vi "MMB.vi"() -> ()   [LabVIEW 2010]
doc: "INTRODUCTION:\nThis program will display a message on the moving message board display based on the user's input. It simulates a moving message board made up of an array of LED's or lights. The user can cause it to display a random pattern of Boolean LED's either turned off or on, a single Boolean LED point scrolling across the display from right to left, a scrolling column of Boolean LED's that can individually be turned on or off, or the message that is entered into the Message control. Any of these options can be repeated as many times as desired by toggling the \"Repeat\" Boolean Control. There is also a \"Milliseconds to Wait\" control, which adjusts the scrolling delay so that the scrolling looks smooth. Foreground and background colors can be changed via color box controls.\n\nDISPLAYING A MESSAGE:\nIf the user chooses to display a message, a configuration file is used which defines how the ASCII characters in the message look. This configuration file can be created with the help of the \"Character Maker.vi\", which allows the user to edit a 17x17 array of Boolean LED's and then generate the key-value pairs to be used in the configuration file to define a given character. The configuration file defines how each character in the \"Message\" box gets displayed. It can be used to make the letters look different (like using a different font) or could be used to make the letters look like something different entirely. For example, you could make the letter \"A\" display a picture of a fish."
uses:
  <vilib>/Utility/config.llb/Read Key (I32).vi
  <vilib>/Utility/config.llb/NI_LVConfig.lvlib
panel:
  in  "LED Off Color":u32(colorbox)
  in  "LED On Color":u32(colorbox)=6291200
  in  "Repeat":bool
  in  "Display Message":bool
  in  "Column":bool
  in  "1 Point":bool
  in  "Random":bool
  in  "stop":bool
  in  "Config Path":path=path "c:/Ed's Files/LabVIEW Files/Moving Message Board/mmb.ini"
  in  "Message":string="The Quick Brown Fox Jumped Over the Lazy Dog"
  in  "Column":bool[](array[boolean])=[TRUE, FALSE, TRUE, FALSE, TRUE, FALSE, TRUE, FALSE, TRUE, FALSE, TRUE, FALSE, TRUE, FALSE, TRUE, FALSE, TRUE]
  in  "1 Point":i32(slide)=8
  in  "Milliseconds to Wait":u32(knob)=50 scale=0.0..1000.0
  out "Array":bool[][](array[boolean])
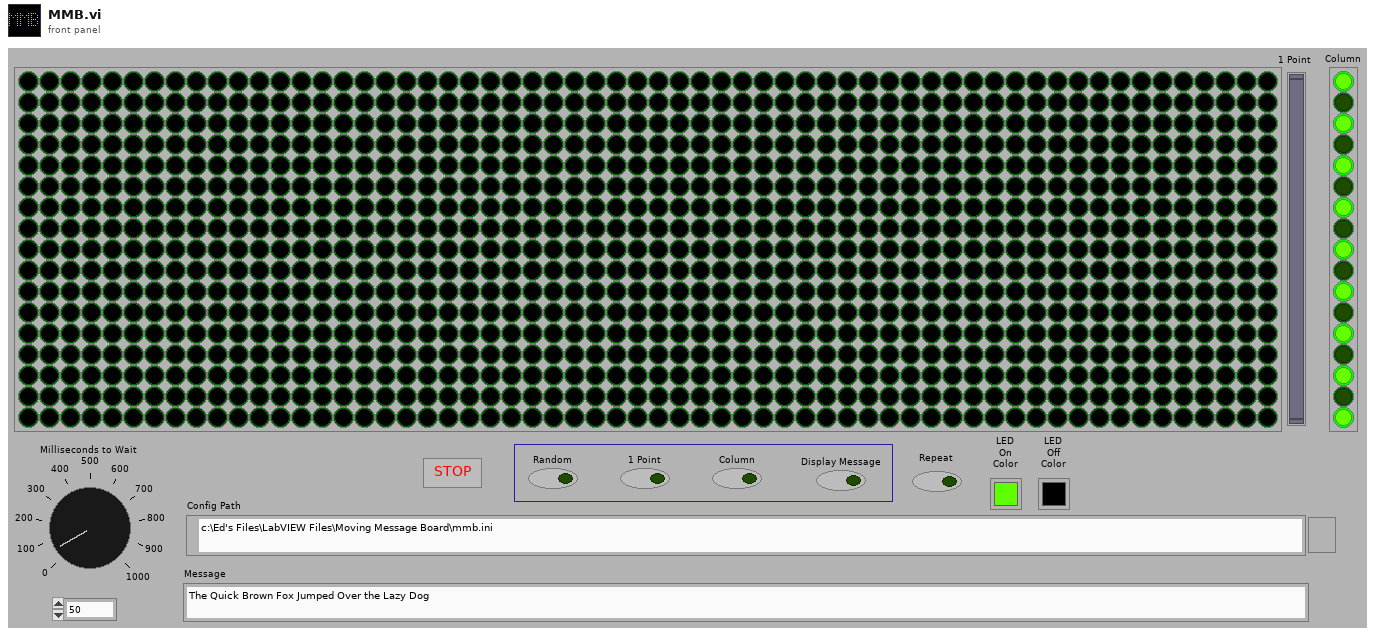
[diagram p1: front panel]
types:
  T1 = cluster{"LED Off Color":u32, "LED Off Color":u32}
  T2 = cluster{"LED On Color":u32, "LED On Color":u32}[]
  T3 = typedef "NI_LVConfig.lvlib/Config Data RefNum.ctl" = refnum<k1>
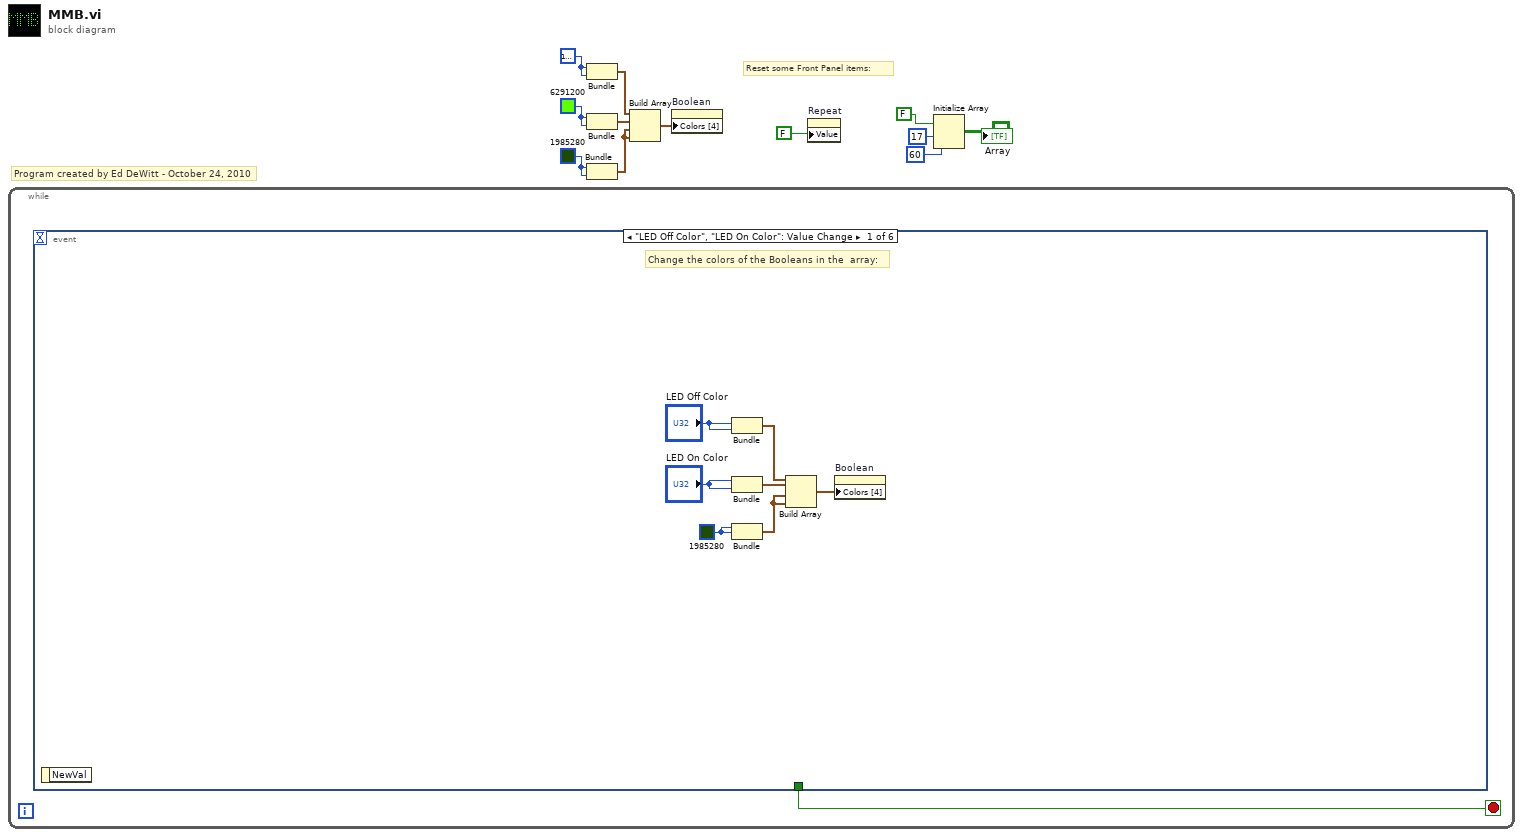
[diagram p0: block diagram]
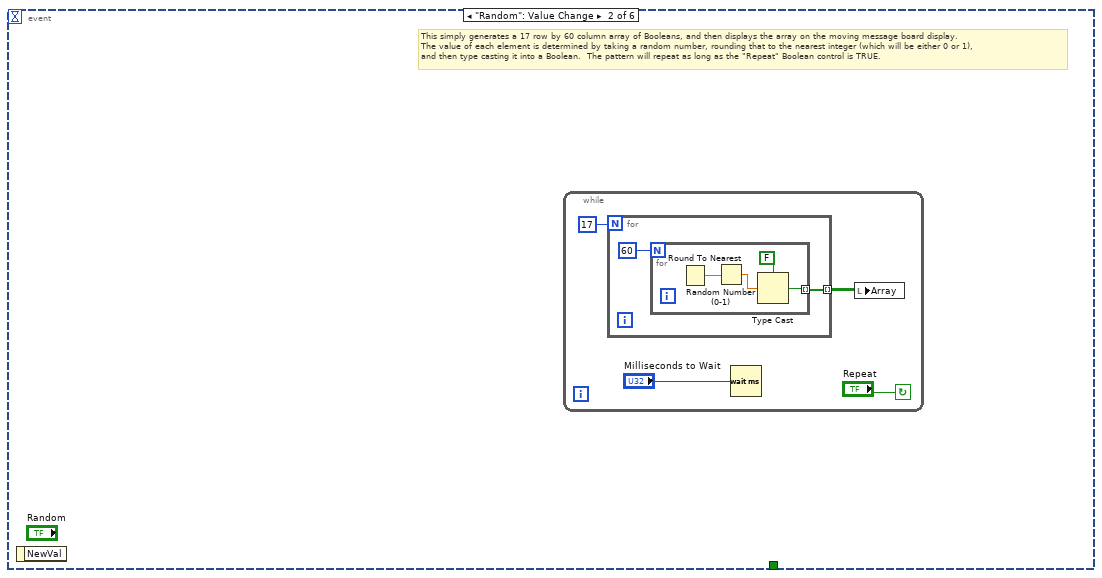
[diagram p2: hidden frame]
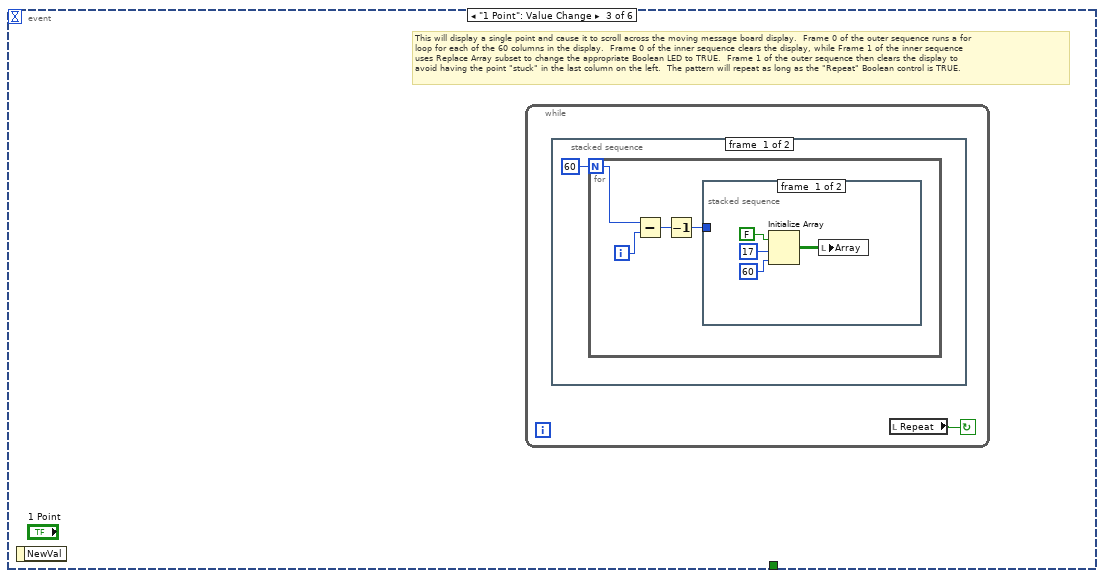
[diagram p3: hidden frame]
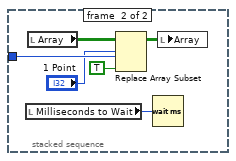
[diagram p4: hidden frame]
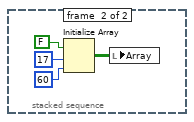
[diagram p5: hidden frame]
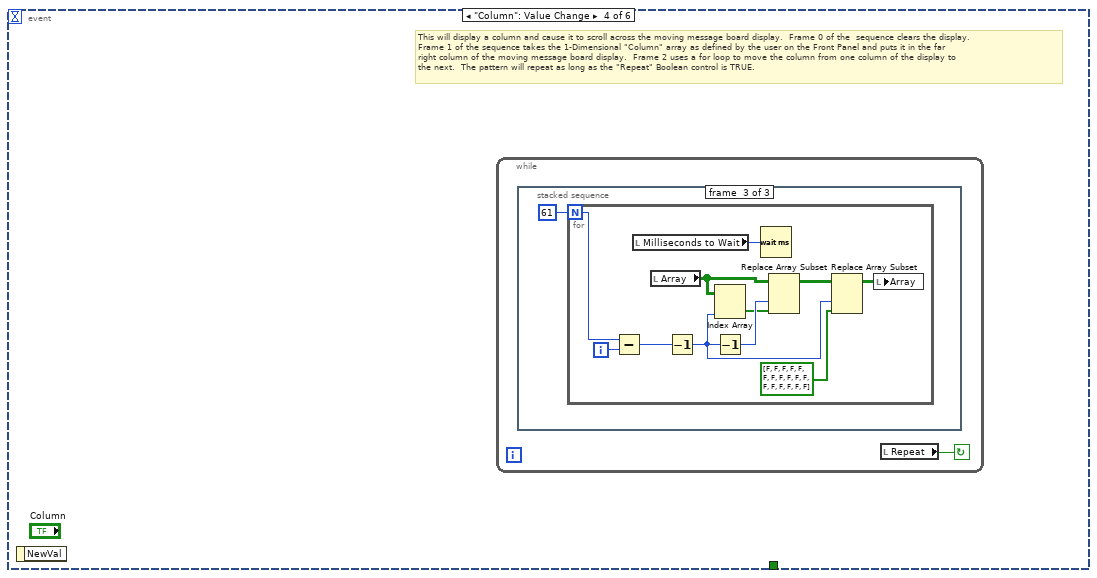
[diagram p6: hidden frame]
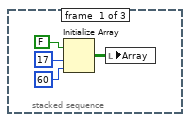
[diagram p7: hidden frame]
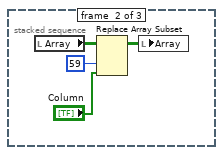
[diagram p8: hidden frame]
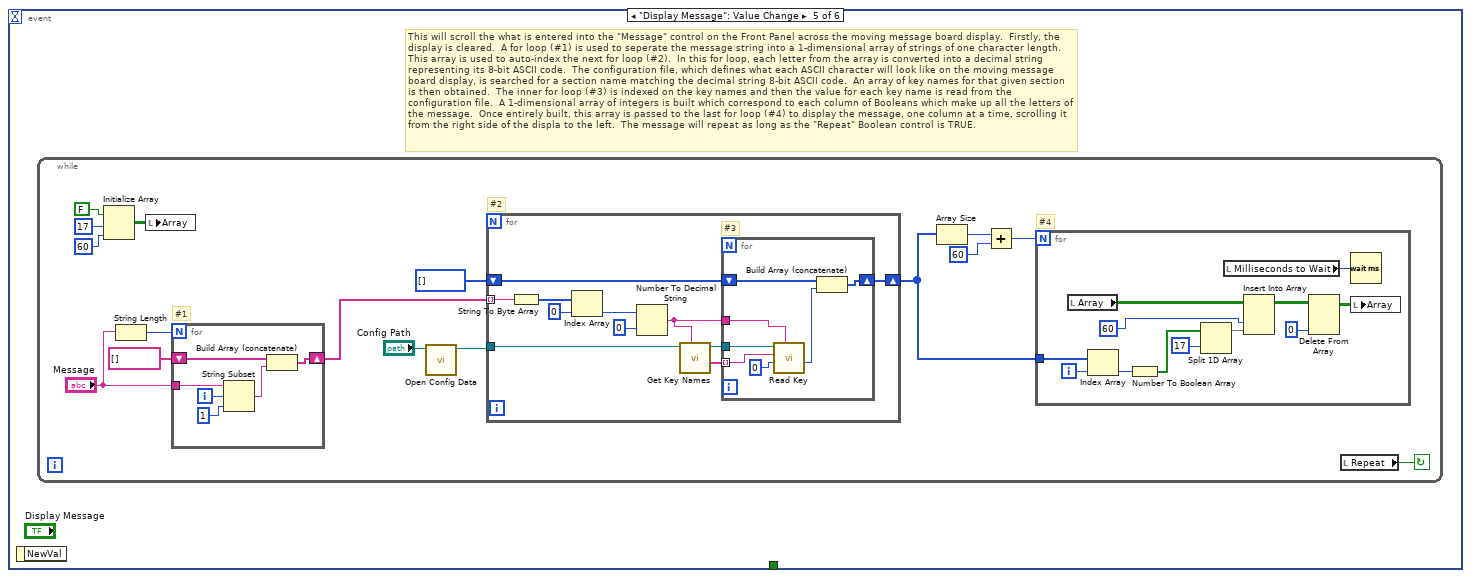
[diagram p9: hidden frame]
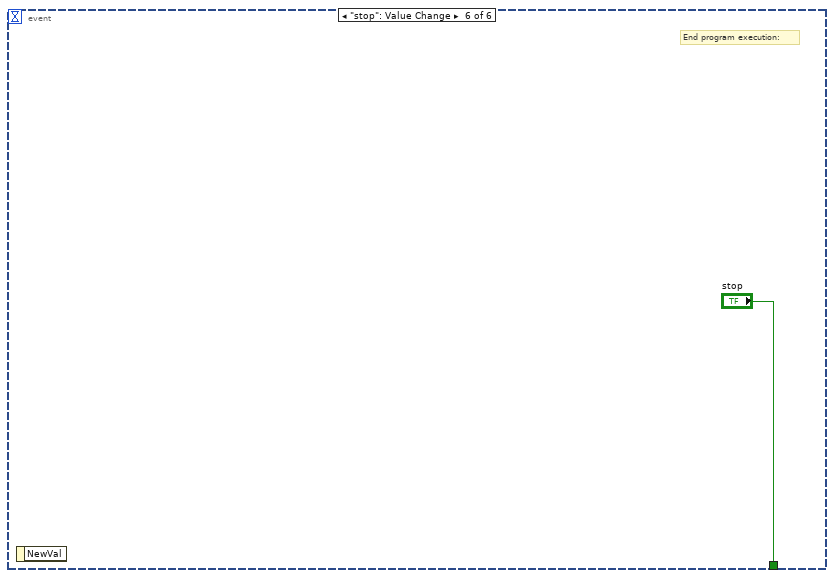
[diagram p10: hidden frame]
diagram:
  w1 = u32 6291200
  w2 = u32 16777222
  w6 = u32 1985280
  # "Program created by Ed DeWitt - October 24, 2010"
  # "Reset some Front Panel items:"
  n1 = while {
    stop <- w13 stop-if-true
    n2 = event shown="[0] \"LED Off Color\", \"LED On Color\": Value Change" {
      selector: _ -> [_ _ _ _ _ _]
      dyn-events: _ -> [_ _ _ _ _ _]
      timeout: _ -> [_ _ _ _ _ _]
      tunnel: [_ _ _ _ _ "stop"] -> w13
      event "LED Off Color", "LED On Color": Value Change {
        w16 = u32 1985280
        # "Change the colors of the Booleans in the  array:"
        n3 = event-data() -> ()  [unwired: 1 in, 1 out]
        n4 = Bundle("LED Off Color"="LED Off Color", "LED Off Color"="LED Off Color") -> (w14:T1)  [unwired: 1 out]
        n5 = Bundle("LED On Color"="LED On Color", "LED On Color"="LED On Color") -> (w20:cluster{"LED On Color":u32, "LED On Color":u32})  [unwired: 1 out]
        n6 = Bundle(w16, w16) -> (w19:cluster{u32, u32})  [unwired: 1 out]
        n7 = Build Array(w14, w20, w19, w19) -> (w17:T2)
        n8 = property on="Boolean" class="Bool (strict)"("Colors [4]"=w17) -> ()  [unwired: 2 in, 2 out]
      }
      event "Random": Value Change {
        # "This simply generates a 17 row by 60 column array of Booleans, and then displays the array on the moving message board display.\nThe value of each element is determined by taking a random number, rounding that to the nearest integer (which will be either 0 or 1),\nand then type casting it into a Boolean.  The pattern will repeat as long as the \"Repeat\" Boolean control is TRUE."
        n9 = event-data() -> ()  [unwired: 1 in, 1 out]
        n10 = while {
          stop <- "Repeat" continue-if-true
          n11 = for {
            N: 17 -> [_]
            tunnel: [w25] -> w23 mode=indexing
            n12 = for {
              N: 60 -> [_]
              tunnel: [w27] -> w25 mode=indexing
              n13 = Random Number (0-1)() -> (number: 0 to 1=w30:dbl)
              n14 = Round To Nearest(number=w30) -> (nearest integer value=w28:dbl)
              n15 = Type Cast(type=FALSE, x=w28) -> (*(type *) &x=w27:bool)
            }
          }
          n16 = Wait (ms)(milliseconds to wait="Milliseconds to Wait") -> ()  [unwired: 1 out]
          n17 = local write "Array"(w23) -> ()
        }
      }
      event "1 Point": Value Change {
        # "This will display a single point and cause it to scroll across the moving message board display.  Frame 0 of the outer sequence runs a for \nloop for each of the 60 columns in the display.  Frame 0 of the inner sequence clears the display, while Frame 1 of the inner sequence\nuses Replace Array subset to change the appropriate Boolean LED to TRUE.  Frame 1 of the outer sequence then clears the display to\navoid having the point \"stuck\" in the last column on the left.  The pattern will repeat as long as the \"Repeat\" Boolean control is TRUE."
        n18 = event-data() -> ()  [unwired: 1 in, 1 out]
        n19 = while {
          stop <- w31 continue-if-true
          n20 = stacked-sequence {
            frame #0 {
              n21 = for {
                N: 60 -> [w36]
                i -> [w35]
                n22 = Subtract(x=w36, y=w35) -> (x-y=w34:i32)
                n23 = Decrement(x=w34) -> (x-1=w33:i32)
                n24 = stacked-sequence {
                  tunnel: w33 -> [_ w45]
                  frame #0 {
                    n25 = Initialize Array(FALSE, 17 ("dimension size"), 60 ("dimension size")) -> (w40:bool[][])
                    n26 = local write "Array"(w40) -> ()
                  }
                  frame #1 {
                    n27 = local read "Milliseconds to Wait"() -> (w42:u32)
                    n28 = local read "Array"() -> (w46:bool[][])
                    n29 = Replace Array Subset(array=w46, new element=TRUE, index (row)="1 Point", index (col)=w45) -> (w43:bool[][])
                    n30 = Wait (ms)(milliseconds to wait=w42) -> ()  [unwired: 1 out]
                    n31 = local write "Array"(w43) -> ()
                  }
                }
              }
            }
            frame #1 {
              n32 = Initialize Array(FALSE, 17 ("dimension size"), 60 ("dimension size")) -> (w47:bool[][])
              n33 = local write "Array"(w47) -> ()
            }
          }
          n34 = local read "Repeat"() -> (w31:bool)
        }
      }
      event "Column": Value Change {
        # "This will display a column and cause it to scroll across the moving message board display.  Frame 0 of the  sequence clears the display.\nFrame 1 of the sequence takes the 1-Dimensional \"Column\" array as defined by the user on the Front Panel and puts it in the far\nright column of the moving message board display.  Frame 2 uses a for loop to move the column from one column of the display to \nthe next.  The pattern will repeat as long as the \"Repeat\" Boolean control is TRUE."
        n35 = event-data() -> ()  [unwired: 1 in, 1 out]
        n36 = while {
          stop <- w51 continue-if-true
          n37 = stacked-sequence {
            frame #0 {
              n38 = Initialize Array(FALSE, 17 ("dimension size"), 60 ("dimension size")) -> (w52:bool[][])
              n39 = local write "Array"(w52) -> ()
            }
            frame #1 {
              n40 = local read "Array"() -> (w59:bool[][])
              n41 = Replace Array Subset(array=w59, new element="Column", index (col)=59 ("disabled index (col)")) -> (w57:bool[][])  [unwired: 1 in]
              n42 = local write "Array"(w57) -> ()
            }
            frame #2 {
              n43 = for {
                N: 61 -> [w68]
                i -> [w67]
                n44 = Subtract(x=w68, y=w67) -> (x-y=w66:i32)
                n45 = local read "Milliseconds to Wait"() -> (w65:u32)
                n46 = local read "Array"() -> (w71:bool[][])
                n47 = Decrement(x=w66) -> (x-1=w63:i32)
                n48 = Index Array(array=w71, index (col)=w63) -> (element=w69:bool[])  [unwired: 1 in]
                n49 = Decrement(x=w63) -> (x-1=w70:i32)
                n50 = Wait (ms)(milliseconds to wait=w65) -> ()  [unwired: 1 out]
                n51 = Replace Array Subset(array=w71, new element=w69, index (col)=w70) -> (w64:bool[][])  [unwired: 1 in]
                n52 = Replace Array Subset(array=w64, new element=bool[] [FALSE, FALSE, FALSE, FALSE, FALSE, FALSE, FALSE, FALSE, FALSE, FALSE, FALSE, FALSE, FALSE, FALSE, FALSE, FALSE, FALSE], index (col)=w63) -> (w61:bool[][])  [unwired: 1 in]
                n53 = local write "Array"(w61) -> ()
              }
            }
          }
          n54 = local read "Repeat"() -> (w51:bool)
        }
      }
      event "Display Message": Value Change {
        # "This will scroll the what is entered into the \"Message\" control on the Front Panel across the moving message board display.  Firstly, the display is cleared.  A for loop (#1) is used to seperate the message string into a 1-dimensional array of strings of one character length.  This array is used to auto-index the next for loop (#2).  In this for loop, each letter from the array is converted into a decimal string representing its 8-bit ASCII code.  The configuration file, which defines what each ASCII character will look like on the moving message board display, is searched for a section name matching the decimal string 8-bit ASCII code.  An array of key names for that given section is then obtained.  The inner for loop (#3) is indexed on the key names and then the value for each key name is read from the configuration file.  A 1-dimensional array of integers is built which correspond to each column of Booleans which make up all the letters of the message.  Once entirely built, this array is passed to the last for loop (#4) to display the message, one column at a time, scrolling it from the right side of the displa to the left.  The message will repeat as long as the \"Repeat\" Boolean control is TRUE."
        n55 = event-data() -> ()  [unwired: 1 in, 1 out]
        n56 = while {
          stop <- w87 continue-if-true
          # "#4"
          # "#2"
          # "#1"
          n57 = Initialize Array(FALSE, 17 ("dimension size"), 60 ("dimension size")) -> (w83:bool[][])
          n58 = String Length(string="Message") -> (length=w80:i32)
          n59 = local write "Array"(w83) -> ()
          n60 = for {
            N: w80 -> [_]
            tunnel: "Message" -> [w123]
            shift-right: [w120] -> w78
            shift-left: string[] [] -> [w119]
            i -> [w122]
            n61 = String Subset(string=w123, offset (0)=w122, length (rest)=1 ("length (rest)")) -> (substring=w118:string)
            n62 = Build Array (concatenate)(w119, w118) -> (w120:string[])
          }
          n63 = call <vilib>:"Open Config Data.vi"("configuration file path"="Config Path") -> ("refnum"=w79:T3)  [unwired: 8 in, 2 out]
          n64 = for {
            tunnel: w79 -> [w110]
            tunnel: w78 -> [w101] mode=indexing
            shift-right: [w107] -> w72
            shift-left: i32[] [] -> [w106]
            # "#3"
            n65 = String To Byte Array(string=w101) -> (unsigned byte array=w102:u8[])
            n66 = Index Array(array=w102, index=0) -> (element=w104:u8)
            n67 = Number To Decimal String(number=w104, width (-)=i16 0) -> (decimal integer string=w100:string)
            n68 = call <vilib>:"Get Key Names.vi"("section"=w100, "refnum"=w110) -> ("key names"=w109:string[], "refnum out"=w108:T3)  [unwired: 1 in, 7 out]
            n69 = for {
              tunnel: w109 -> [w116] mode=indexing
              tunnel: w108 -> [w115]
              shift-right: [w111] -> w107
              shift-left: w106 -> [w112]
              tunnel: w100 -> [w117]
              n70 = call-poly <vilib>:"Read Key.vi"("section"=w117, "default value"=0, "key"=w116, "refnum"=w115) -> ("value"=w114:i32)  [unwired: 1 in, 6 out]
              n71 = Build Array (concatenate)(w112, w114) -> (w111:i32[])
            }
          }
          n72 = Array Size(array=w72) -> (size(s)=w73:i32)
          n73 = Add(x=w73, y=60) -> (x+y=w74:i32)
          n74 = for {
            N: w74 -> [_]
            tunnel: w72 -> [w88]
            i -> [w98]
            n75 = local read "Array"() -> (w99:bool[][])
            n76 = Index Array(array=w88, index=w98) -> (element=w97:i32)
            n77 = Number To Boolean Array(number=w97) -> (Boolean array=w92:bool[])
            n78 = Split 1D Array(array=w92, index=17) -> (first subarray=w90:bool[])  [unwired: 1 out]
            n79 = local read "Milliseconds to Wait"() -> (w89:u32)
            n80 = Insert Into Array(array=w99, index (col)=60 ("disabled index (col)"), new element=w90) -> (w95:bool[][])  [unwired: 1 in]
            n81 = Delete From Array(array=w95, index (col)=0 ("disabled index (col)")) -> (array with subset deleted=w93:bool[][])  [unwired: 2 in, 1 out]
            n82 = Wait (ms)(milliseconds to wait=w89) -> ()  [unwired: 1 out]
            n83 = local write "Array"(w93) -> ()
          }
          n84 = local read "Repeat"() -> (w87:bool)
        }
      }
      event "stop": Value Change {
        # "End program execution:"
        n85 = event-data() -> ()  [unwired: 1 in, 1 out]
      }
    }
  }
  n86 = Bundle(w2, w2) -> (w7:cluster{u32, u32})  [unwired: 1 out]
  n87 = Bundle(w1, w1) -> (w3:cluster{u32, u32})  [unwired: 1 out]
  n88 = Bundle(w6, w6) -> (w4:cluster{u32, u32})  [unwired: 1 out]
  n89 = Build Array(w7, w3, w4, w4) -> (w5:cluster{u32, u32}[])
  n90 = property on="Boolean" class="Bool (strict)"("Colors [4]"=w5) -> ()  [unwired: 2 in, 2 out]
  n91 = property on="Repeat" class="Bool (strict)"("Value"=FALSE) -> ()  [unwired: 2 in, 2 out]
  n92 = Initialize Array(FALSE, 17 ("dimension size"), 60 ("dimension size")) -> (→"Array":bool[][])
